vi "XBee_PC.vi"() -> ()   [LabVIEW 2015]
uses:
  <vilib>/Instr/_visa.llb/VISA Configure Serial Port (Instr).vi
panel:
  in  "Transmit Data":string="XBee模組測試"
  out "Receive Data":string
  out "Z-Axis":dbl(slide) scale=-2.0..2.0
  out "Y-Axis":dbl(slide) scale=-2.0..2.0
  out "X-Axis":dbl(slide) scale=-2.0..2.0
  out "Button":bool
  in  "LED":bool[](array[boolean])=[FALSE, FALSE, FALSE, FALSE]
  in  "XBee Address":u64[](array[numeric])=[5526146529826789, 5526146529826775] format="%016x"
  in  "stop":bool
  # "XBeeNo.1   0013A20040E317E5"
  # "XBeeNO.2  0013A20040E317D7"
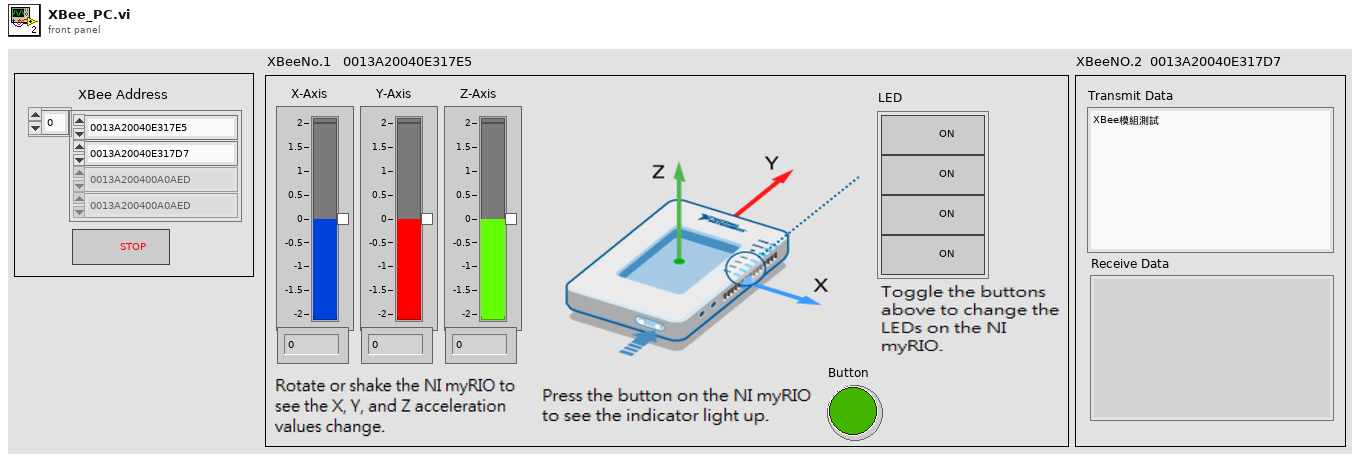
[diagram p1: front panel]
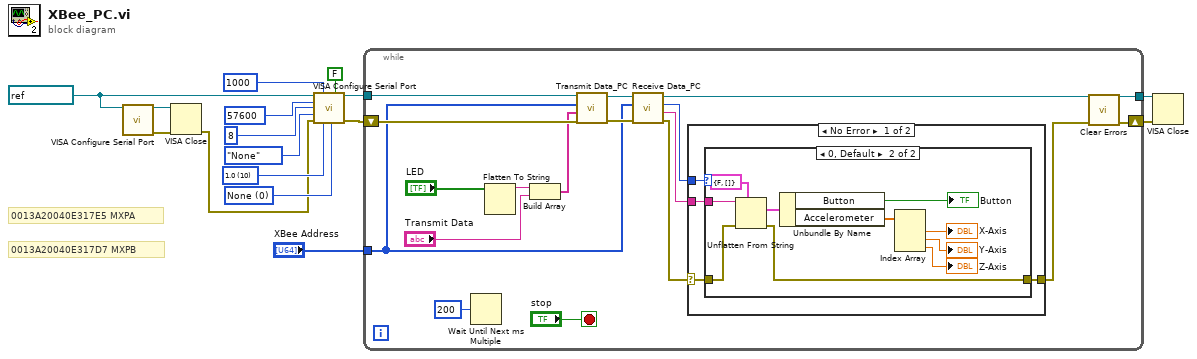
[diagram p0: block diagram]
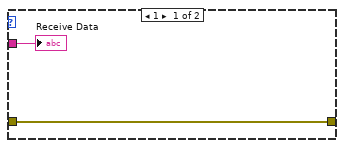
[diagram p2: hidden frame]
diagram:
  w2 = refnum<visa-resource-name> "COM5" ("VISA resource name")
  w13 = u16 10 items=["1.0"=10, "1.5"=15, "2.0"=20] ("stop bits (10: 1 bit)")
  w14 = u16 0 items=["None", "XON/XOFF", "RTS/CTS", "XON/XOFF & RTS/CTS", "DTR/DSR", "XON/XOFF & DTR/DSR"] ("flow control (0:none)")
  # "0013A20040E317D7 MXPB"
  # "0013A20040E317E5 MXPA"
  n1 = call-poly "VISA Configure Serial Port"("VISA resource name"=w2) -> ("VISA resource name out"=w3:refnum<visa-resource-name>, "error out"=w4:errorcluster)  [unwired: 13 in]
  n2 = VISA Close(VISA resource name=w3, error in (no error)=w4) -> (error out=w1:errorcluster)
  n3 = call-poly "VISA Configure Serial Port"("VISA resource name"=w2, "timeout (10sec)"=u32 1000, "Enable Termination\nChar (T)"=FALSE ("Enable Termination\nChar (T)"), "baud rate (9600)"=u32 57600, "data bits (8)"=u16 8, "parity (0:none)"=enum16{"None", "Odd", "Even", "Mark", "Space"}."None", "error in (no error)"=w1, "stop bits (10: 1 bit)"=w13, "flow control (0:none)"=w14) -> ("VISA resource name out"=w10:refnum<visa-resource-name>, "error out"=w9:errorcluster)  [unwired: 5 in]
  n4 = while {
    tunnel: w10 -> [w29]
    shift-right: [w17] -> w8
    shift-left: w9 -> [w30]
    tunnel: "XBee Address" -> [w27]
    tunnel: [w28] -> w7
    stop <- "stop" stop-if-true
    n5 = Wait Until Next ms Multiple(millisecond multiple=u32 200) -> ()  [unwired: 1 out]
    n6 = Flatten To String(anything="LED") -> (data string=w21:string)  [unwired: 3 in, 2 out]
    n7 = Build Array(w21, "Transmit Data") -> (w25:string[])
    n8 = call "Transmit Data_PC.vi"("error in (no error)"=w30, "Transmit Data"=w25, "Address"=w27, "VISA resource name"=w29) -> ("error out"=w31:errorcluster, "VISA resource name out"=w32:refnum<visa-resource-name>)  [unwired: 6 in]
    n9 = call "Receive Data_PC.vi"("error in (no error)"=w31, "Address"=w27, "VISA Refnum in"=w32) -> ("error out"=w19:errorcluster, "Receive Data"=w23:string, "Index Data"=w24:i32, "VISA Refnum out"=w28:refnum<visa-resource-name>)  [unwired: 5 in]
    n10 = case shown="No Error" w19 {
      selector: w19 -> [w35 w50]
      tunnel: w24 -> [w37 _]
      tunnel: w23 -> [w36 _]
      tunnel: [w34 w50] -> w18
      frame No Error {
        n11 = case shown="0, Default" w37 {
          tunnel: w36 -> [w39 w49]
          tunnel: w35 -> [w38 w41]
          tunnel: [w38 w40] -> w34
          frame 1 {
            "Receive Data" <- w39
          }
          frame 0, Default {
            n12 = Unflatten From String(type=cluster{"Button":bool, "Accelerometer":dbl[]} {"Button"=FALSE, "Accelerometer"=[]}, binary string=w49, error in (no error)=w41) -> (value=w47:cluster{"Button":bool, "Accelerometer":dbl[]}, error out=w40:errorcluster)  [unwired: 2 in, 1 out]
            n13 = Unbundle By Name(w47) -> ("Button"=→"Button":bool, "Accelerometer"=w45:dbl[])
            n14 = Index Array(array=w45) -> (element #1=→"X-Axis":dbl, element #2=→"Y-Axis":dbl, element #3=→"Z-Axis":dbl)  [unwired: 3 in]
          }
        }
      }
      frame Error {
      }
    }
    n15 = call <vilib>:"Clear Errors.vi"("error in (no error)"=w18) -> ("error out"=w17:errorcluster)  [unwired: 5 in, 1 out]
  }
  n16 = VISA Close(VISA resource name=w7, error in (no error)=w8) -> ()  [unwired: 1 out]
